vi "Update.vi"(8 "error in (no error)":errorcluster, 9 "Digital Outputs":T1, 10 "Analog Outputs":T2, 11 "PXI in":refnum<class "PXI.lvclass">) -> (0 "error out":errorcluster, 1 "Digital Inputs":T1, 2 "Analog Inputs":T2, 3 "PXI out":refnum<class "PXI.lvclass">)   [LabVIEW 2011, in "PXI.lvclass"]
uses:
  PXI.lvclass
  Controls/Analog Values.ctl
  Controls/Digital Values.ctl
  PXI.lvclass/PXI.ctl
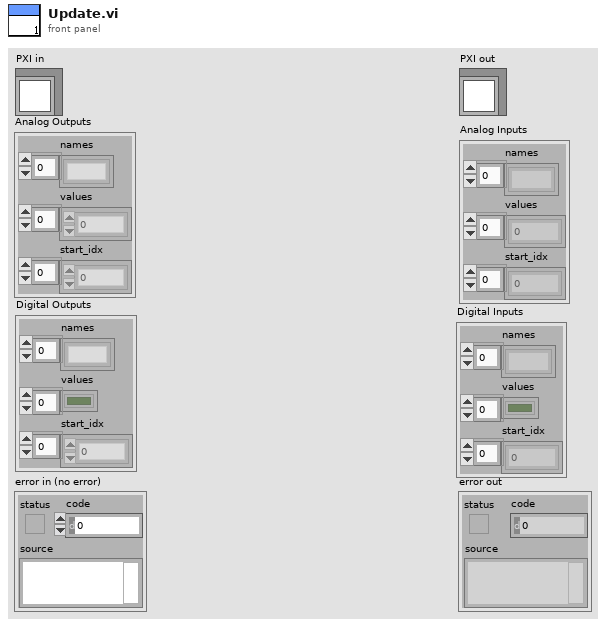
[diagram p1: front panel]
types:
  T1 = typedef "Digital Values.ctl" = cluster{"names":string[], "values":bool[], "start_idx":i32[]}
  T2 = typedef "Analog Values.ctl" = cluster{"names":string[], "values":dbl[], "start_idx":i32[]}
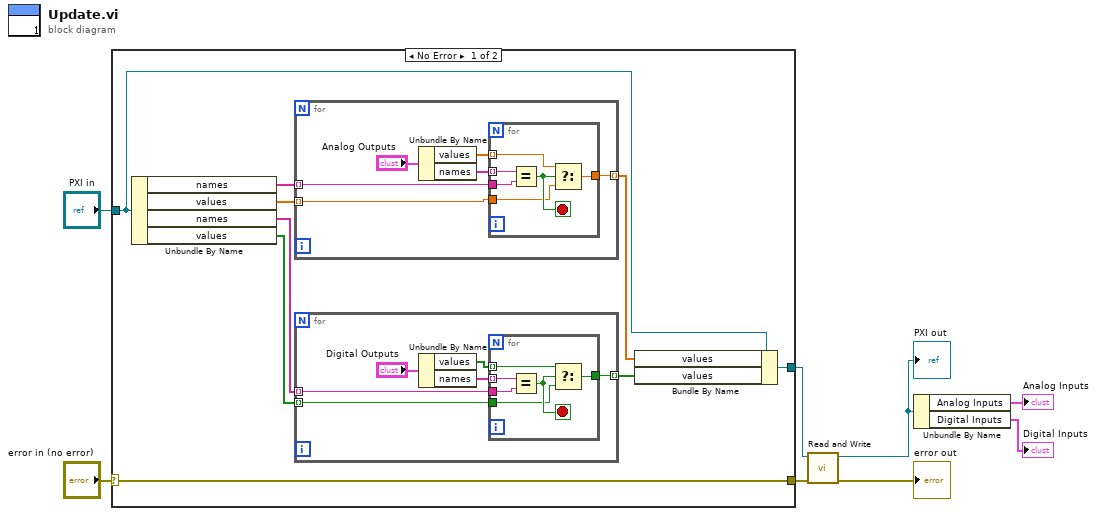
[diagram p0: block diagram]
diagram:
  n1 = case shown="No Error" "error in (no error)" {
    selector: "error in (no error)" -> [w17 w43]
    tunnel: [w17 w43] -> w5
    tunnel: [w9 w42] -> w6
    tunnel: "PXI in" -> [w12 w42]
    frame No Error {
      n2 = Unbundle By Name(w12) -> ("names"=w13:string[], "values"=w14:dbl[], "names"=w16:string[], "values"=w15:bool[])
      n3 = for {
        tunnel: [w35] -> w10 mode=indexing
        tunnel: w14 -> [w32] mode=indexing
        tunnel: w13 -> [w31] mode=indexing
        n4 = Unbundle By Name("Analog Outputs") -> ("values"=w30:dbl[], "names"=w33:string[])
        n5 = for {
          tunnel: w31 -> [w39]
          tunnel: w32 -> [w38]
          tunnel: [w41] -> w35
          tunnel: w33 -> [w37] mode=indexing
          tunnel: w30 -> [w36] mode=indexing
          stop <- w40 stop-if-true
          n6 = Equal?(x=w37, y=w39) -> (x = y?=w40:bool)
          n7 = Select(t=w36, s=w40, f=w38) -> (s? t:f=w41:dbl)
        }
      }
      n8 = for {
        tunnel: [w23] -> w11 mode=indexing
        tunnel: w15 -> [w22] mode=indexing
        tunnel: w16 -> [w21] mode=indexing
        n9 = Unbundle By Name("Digital Outputs") -> ("values"=w19:bool[], "names"=w18:string[])
        n10 = for {
          tunnel: w21 -> [w27]
          tunnel: w22 -> [w26]
          tunnel: [w29] -> w23
          tunnel: w18 -> [w25] mode=indexing
          tunnel: w19 -> [w24] mode=indexing
          stop <- w28 stop-if-true
          n11 = Equal?(x=w25, y=w27) -> (x = y?=w28:bool)
          n12 = Select(t=w24, s=w28, f=w26) -> (s? t:f=w29:bool)
        }
      }
      n13 = Bundle By Name(cluster=w12, "values"=w10, "values"=w11) -> (w9:refnum<class "PXI.lvclass">)
    }
    frame Error {
    }
  }
  n14 = call "Read and Write.vi"("error in (no error)"=w5, "PXI in"=w6) -> ("error out"=→"error out":errorcluster, "PXI out"=w3:refnum<class "PXI.lvclass">)  [unwired: 8 in]
  "PXI out" <- w3
  n15 = Unbundle By Name(w3) -> ("Analog Inputs"=→"Analog Inputs":T2, "Digital Inputs"=→"Digital Inputs":T1)
